vi "Autonomous Independent.vi"   [LabVIEW 2015]
doc: "This VI is called when autonomous begins, and will automatically be terminated when autonomous ends. You can carry out timed or sensor driven robot movement independently without needing to return to the caller."
uses:
  Team Code/Periodic Task/Auto/Auto_Selection.ctl
  <vilib>/Rock Robotics/WPI/Utilities/WPI_GetSetVariantRefNum.vi
  <vilib>/Rock Robotics/Network Tables/NT Read String.vi
  <vilib>/Rock Robotics/Network Tables/NT Write Numeric Array.vi
  <vilib>/Rock Robotics/Network Tables/NT Read Number.vi
  <vilib>/Rock Robotics/Network Tables/NT Read Boolean.vi
  Team Code/Global_Var/Drive_Global.vi
  Team Code/Periodic Task/Auto/Auto_Global.vi
panel:
  # "Be sure to right-click and choose Data Operations>>Make Current Value default if you want to save the array values with the VI"
types:
  T1 = typedef "WPI_JoystickDevRef.ctl" = cluster{"Device":T2}
  T2 = typedef "WPI_JoystickDeviceEnum.ctl" = enum16{"USB 0", "USB 1", "USB 2", "USB 3", "USB 4", "USB 5"}
  T3 = typedef "Auto_Selection.ctl" = enum16{"Low Bar", "Rough Terrain", "Rock Wall", "Ramparts", "Moat", "Cheval de Frise", "Portcullis", "None", "One  Ball", "Shoot"}
  T4 = enum16{"Standard", "Momentary Falling", "Momentary Rising", "Momentary Falling and Rising"}
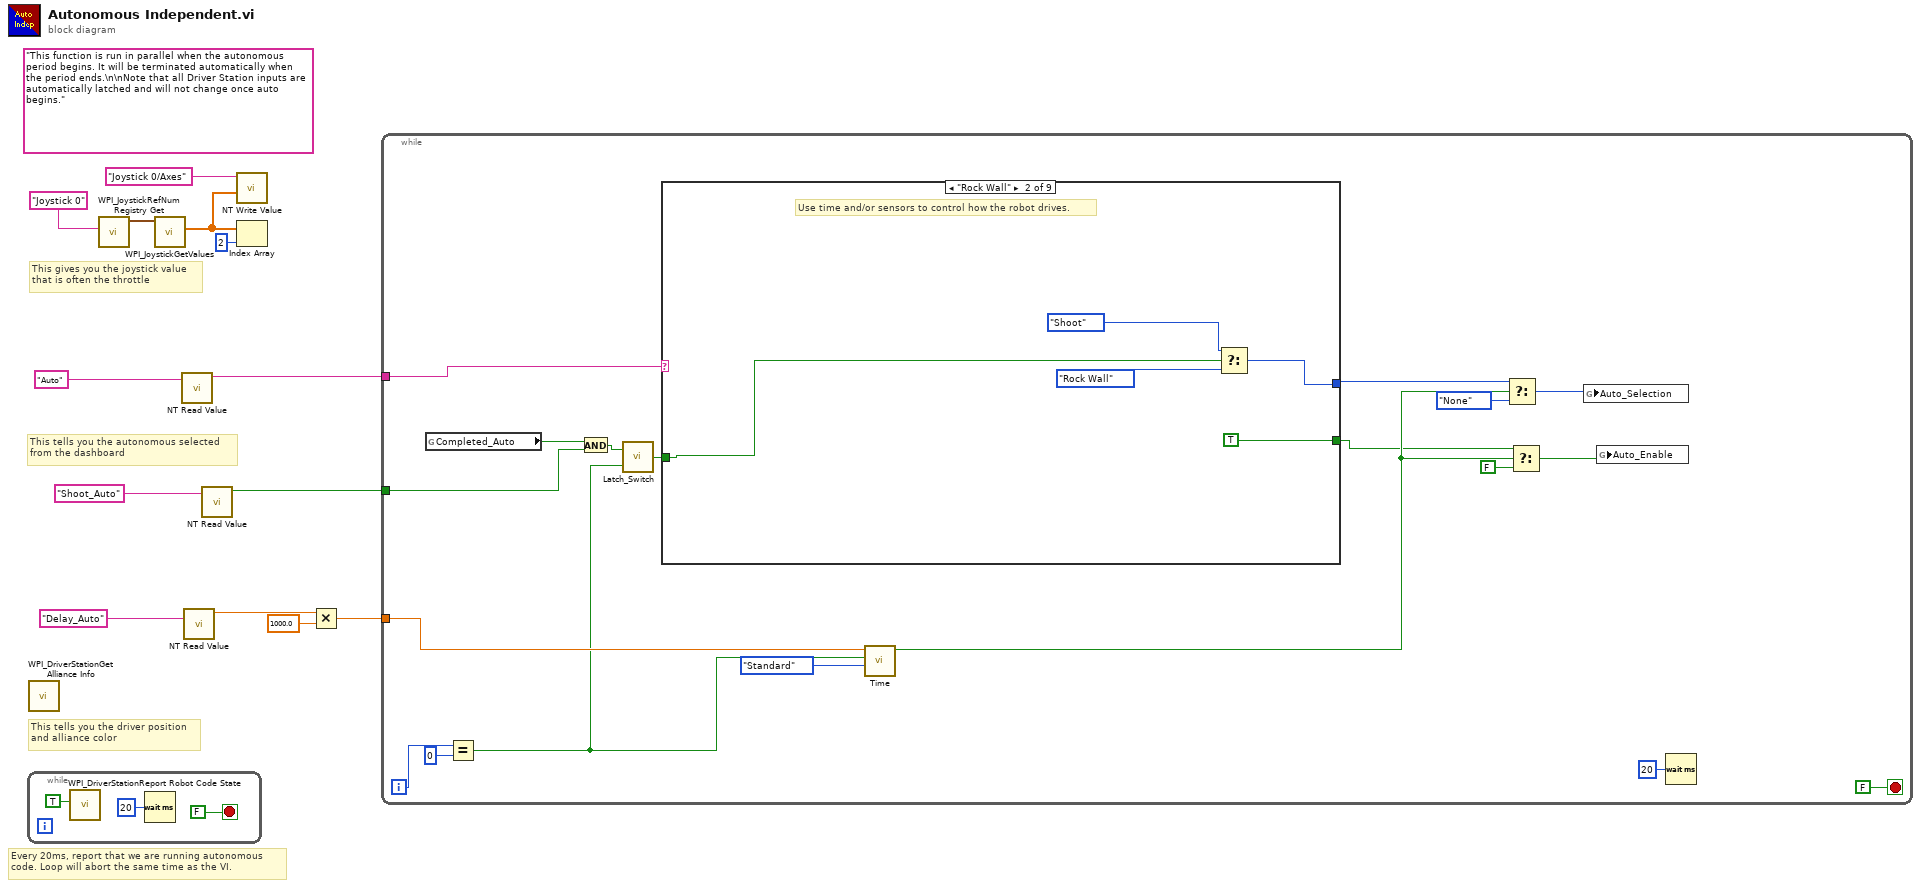
[diagram p0: block diagram]
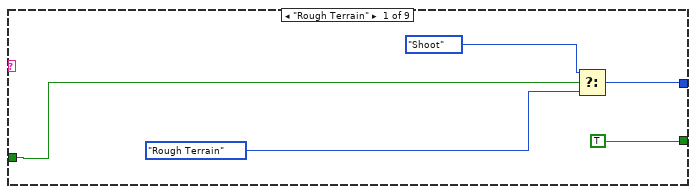
[diagram p2: hidden frame]
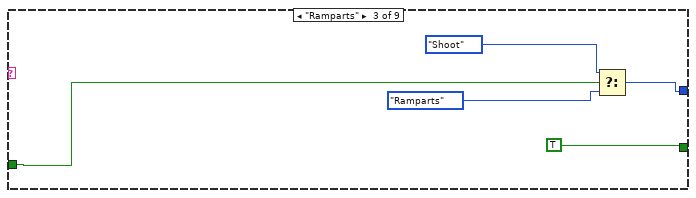
[diagram p3: hidden frame]
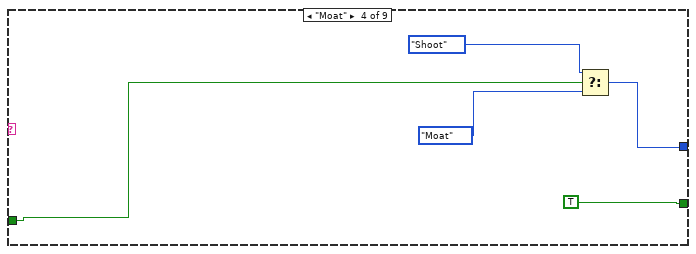
[diagram p4: hidden frame]
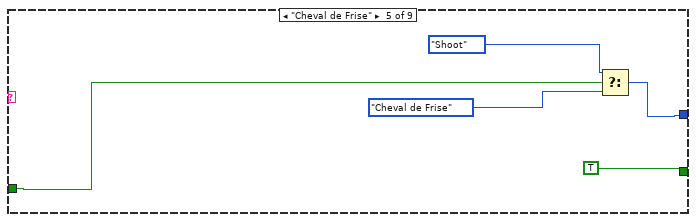
[diagram p5: hidden frame]
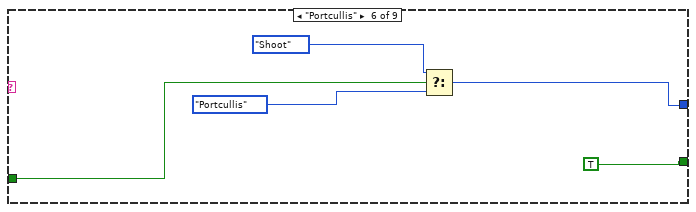
[diagram p6: hidden frame]
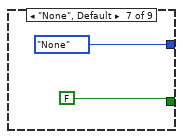
[diagram p7: hidden frame]
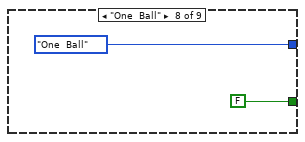
[diagram p8: hidden frame]
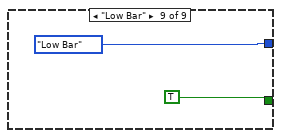
[diagram p9: hidden frame]
diagram:
  (unwired) "This function is run in parallel when the autonomous period begins. It will be terminated automatically when the period ends.\n\nNote that all Driver Station inputs are automatically latched and will not change once auto begins."
  # "This tells you the autonomous selected\nfrom the dashboard"
  # "Every 20ms, report that we are running autonomous\ncode. Loop will abort the same time as the VI."
  # "This gives you the joystick value\nthat is often the throttle"
  # "This tells you the driver position\nand alliance color"
  n1 = while {
    stop <- FALSE stop-if-true
    n2 = call <vilib>:"WPI_DriverStationReport Robot Code State.vi"("Autonomous"=TRUE) -> ()  [unwired: 10 in, 1 out]
    n3 = Wait (ms)(milliseconds to wait=u32 20) -> ()  [unwired: 1 out]
  }
  n4 = call <vilib>:"WPI_DriverStationGet Alliance Info.vi"() -> ()  [unwired: 12 out]
  n5 = call <vilib>:"WPI_JoystickRefNum Registry Get.vi"("refnum name"="Joystick 0") -> ("JoystickDevRef"=w12:T1)  [unwired: 1 in, 9 out]
  n6 = call <vilib>:"WPI_JoystickGetValues.vi"("JoystickDevRef"=w12) -> ("Axes"=w9:dbl[])  [unwired: 6 in, 4 out]
  n7 = call-poly <vilib>:"NT Read Value.vi"("Name"="Auto") -> ("String"=w7:string)  [unwired: 9 in, 1 out]
  n8 = call-poly <vilib>:"NT Read Value.vi"("Name"="Delay_Auto") -> ("Numeric"=w5:dbl)  [unwired: 9 in, 1 out]
  n9 = call-poly <vilib>:"NT Read Value.vi"("Name"="Shoot_Auto") -> ("Boolean"=w1:bool)  [unwired: 9 in, 1 out]
  n10 = call-poly <vilib>:"NT Write Value.vi"("Numeric Array"=w9, "Name"="Joystick 0/Axes") -> ()  [unwired: 9 in, 1 out]
  n11 = Index Array(array=w9, index=2) -> ()  [unwired: 1 out]
  n12 = Multiply(x=w5, y=1000.0) -> (x*y=w3:dbl)
  n13 = while {
    tunnel: w7 -> [w35]
    tunnel: w3 -> [w29]
    tunnel: w1 -> [w20]
    i -> [w31]
    stop <- FALSE stop-if-true
    # "Use time and/or sensors to control how the robot drives."
    n14 = global read "Drive_Global.vi" "Completed_Auto"() -> (w21:bool)
    n15 = Equal?(x=w31, y=0) -> (x = y?=w17:bool)
    n16 = And(x=w21, y=w20) -> (x .and. y?=w19:bool)
    n17 = call "Latch_Switch.vi"("Reset"=w17, "In"=w19) -> ("Out"=w18:bool)
    n18 = case shown="\"Rock Wall\"" w35 {
      tunnel: [w39 w42 w47 w52 w57 w62 Auto_Selection."None" ("Auto_Selection") Auto_Selection."One  Ball" ("Auto_Selection") Auto_Selection."Low Bar" ("Auto_Selection")] -> w25
      tunnel: [TRUE TRUE TRUE TRUE TRUE TRUE FALSE FALSE TRUE] -> w26
      tunnel: w18 -> [w36 w41 w46 w51 w56 w61 _ _ _]
      frame "Rough Terrain" {
        n19 = Select(t=Auto_Selection."Shoot" ("Auto_Selection"), s=w36, f=Auto_Selection."Rough Terrain" ("Auto_Selection")) -> (s? t:f=w39:T3)
      }
      frame "Rock Wall" {
        n20 = Select(t=Auto_Selection."Shoot" ("Auto_Selection"), s=w41, f=Auto_Selection."Rock Wall" ("Auto_Selection")) -> (s? t:f=w42:T3)
      }
      frame "Ramparts" {
        n21 = Select(t=Auto_Selection."Shoot" ("Auto_Selection"), s=w46, f=Auto_Selection."Ramparts" ("Auto_Selection")) -> (s? t:f=w47:T3)
      }
      frame "Moat" {
        n22 = Select(t=Auto_Selection."Shoot" ("Auto_Selection"), s=w51, f=Auto_Selection."Moat" ("Auto_Selection")) -> (s? t:f=w52:T3)
      }
      frame "Cheval de Frise" {
        n23 = Select(t=Auto_Selection."Shoot" ("Auto_Selection"), s=w56, f=Auto_Selection."Cheval de Frise" ("Auto_Selection")) -> (s? t:f=w57:T3)
      }
      frame "Portcullis" {
        n24 = Select(t=Auto_Selection."Shoot" ("Auto_Selection"), s=w61, f=Auto_Selection."Portcullis" ("Auto_Selection")) -> (s? t:f=w62:T3)
      }
      frame "None", Default {
      }
      frame "One  Ball" {
      }
      frame "Low Bar" {
      }
    }
    n25 = call "Time.vi"("Configuration"=T4."Standard", "Reset"=w17, "Time_Limit  (ms)"=w29) -> ("Time_Met"=w27:bool)  [unwired: 8 in]
    n26 = Select(t=w25, s=w27, f=Auto_Selection."None") -> (s? t:f=w34:T3)
    n27 = Select(t=w26, s=w27, f=FALSE) -> (s? t:f=w22:bool)
    n28 = global write "Auto_Global.vi" "Auto_Selection"(w34) -> ()
    n29 = global write "Auto_Global.vi" "Auto_Enable"(w22) -> ()
    n30 = Wait (ms)(milliseconds to wait=u32 20) -> ()  [unwired: 1 out]
  }
